vi "to string.vi"(8 "error in":errorcluster, 11 "TDMS datalogger configuration in":refnum<class "TDMS datalogger configuration.lvclass">) -> (0 "error out":errorcluster, 1 "data":string, 2 "version":string, 3 "TDMS datalogger configuration out":refnum<class "TDMS datalogger configuration.lvclass">)   [LabVIEW 2015, in "TDMS datalogger configuration.lvclass"]
doc: "Provides an interface for saving a module configuration to a file or other serialized data source. It is recommended that all children of this class store data in two sets--data required for its own initialization, and any data required for parent initialization--and that each implementation uses the <b>Call Parent Method</b> primitive to serialize parent information."
uses:
  TDMS datalogger configuration.lvclass
  TDMS datalogger configuration.lvclass/TDMS datalogger configuration.ctl
  <vilib>/NI/Tag Bus Module Framework/module configuration/TBM module configuration.lvclass
  <vilib>/NI/Configuration Framework/serializable configuration/NISE_CEF_serializable configuration.lvclass
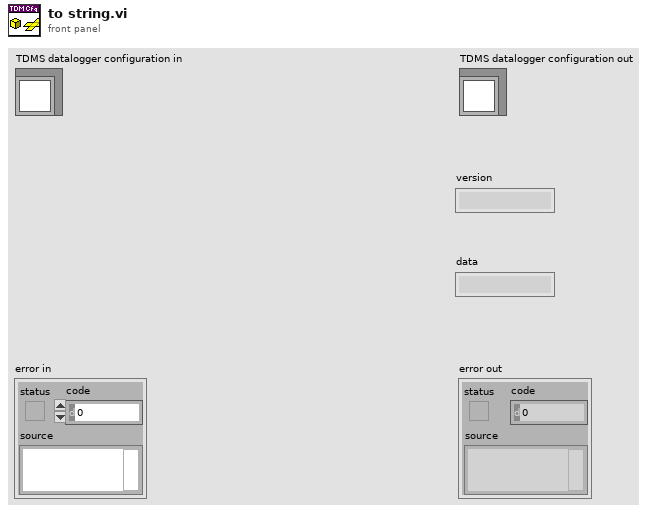
[diagram p1: front panel]
types:
  T1 = typedef "LogRotate.lvclass/options.ctl" = cluster{"max file size (bytes)":i64, "rotate count":u32, "max age (days)":dbl, "No archive dir":bool, "Archive dir":path}
  T2 = typedef "TDMS datalogger configuration.lvclass/Logging Type.ctl" = enum16{"Continuous", "Finite"}
  T3 = typedef "TDMS datalogger configuration.lvclass/Trigger Type.ctl" = enum16{"None", "Start"}
  T4 = typedef "TDMS datalogger configuration.lvclass/Edge Direction.ctl" = enum16{"Rising", "Falling"}
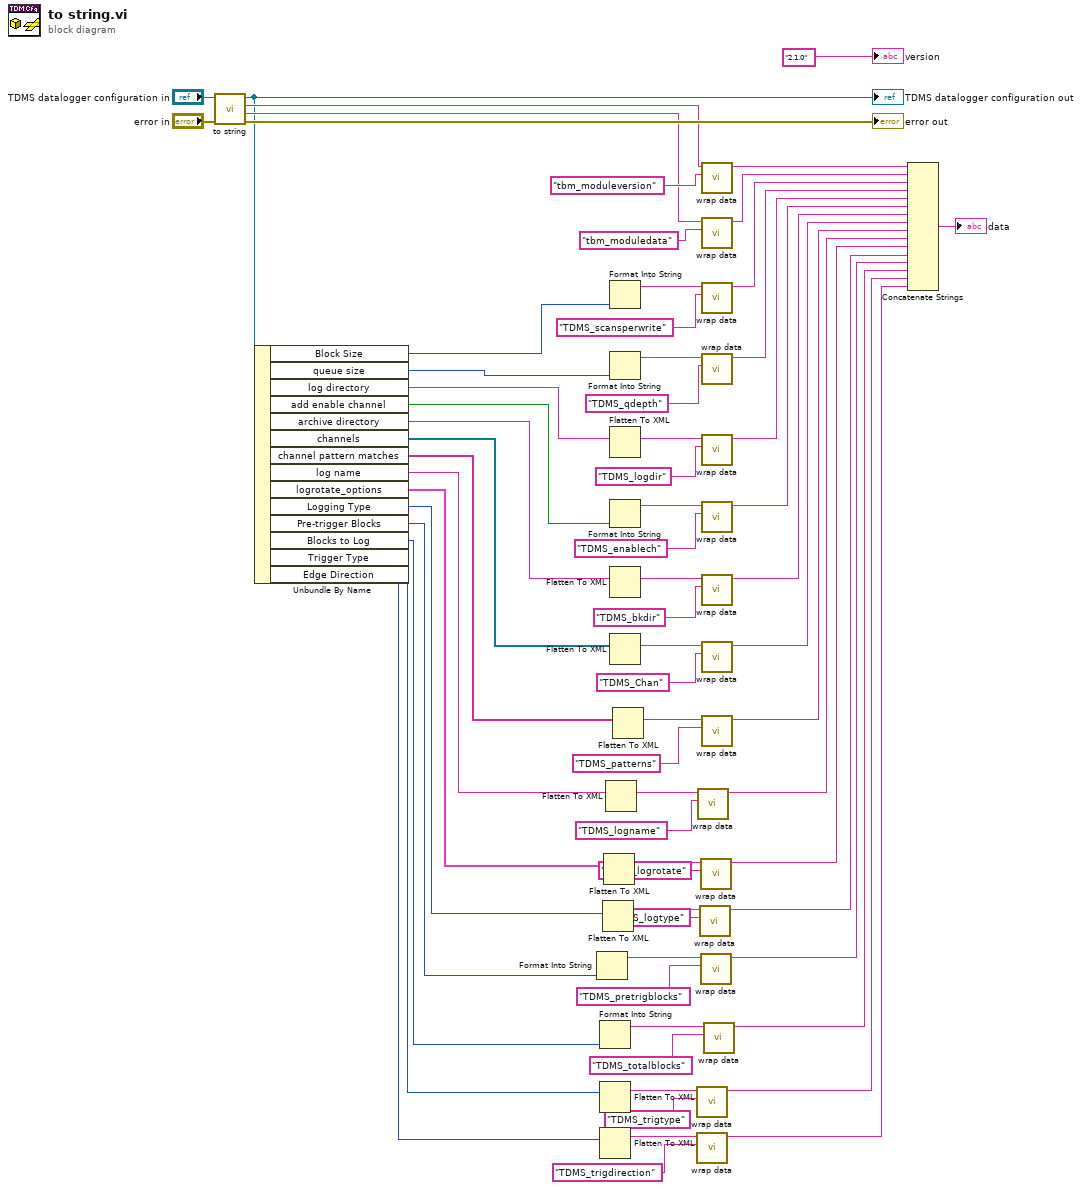
[diagram p0: block diagram]
diagram:
  n1 = call-parent "to string.vi"("error in"="error in", "module configuration in"="TDMS datalogger configuration in") -> ("error out"=→"error out":errorcluster, "data"=w62:string, "version"=w63:string, "module configuration out"=w58:refnum<class "TDMS datalogger configuration.lvclass">)  [unwired: 6 in]
  "TDMS datalogger configuration out" <- w58
  n2 = Unbundle By Name(w58) -> ("Block Size"=w54:u16, "queue size"=w55:u16, "log directory"=w30:string, "add enable channel"=w56:bool, "archive directory"=w29:string, "channels"=w57:refnum<class "TBM channel.lvclass">[], "channel pattern matches"=w35:string[], "log name"=w26:string, "logrotate_options"=w24:T1, "Logging Type"=w18:T2, "Pre-trigger Blocks"=w15:i32, "Blocks to Log"=w12:i32, "Trigger Type"=w9:T3, "Edge Direction"=w6:T4)
  n3 = Format Into String(w15) -> (resulting string=w16:string)  [unwired: 3 in, 1 out]
  n4 = Format Into String(w12) -> (resulting string=w14:string)  [unwired: 3 in, 1 out]
  n5 = Flatten To XML(anything=w9) -> (xml string=w11:string)
  n6 = Flatten To XML(anything=w6) -> (xml string=w8:string)
  n7 = Flatten To XML(anything=w18) -> (xml string=w19:string)
  n8 = Flatten To XML(anything=w24) -> (xml string=w23:string)
  n9 = Flatten To XML(anything=w26) -> (xml string=w27:string)
  n10 = Format Into String(w54) -> (resulting string=w53:string)  [unwired: 3 in, 1 out]
  n11 = Format Into String(w55) -> (resulting string=w51:string)  [unwired: 3 in, 1 out]
  n12 = Flatten To XML(anything=w30) -> (xml string=w49:string)
  n13 = Format Into String(w56) -> (resulting string=w48:string)  [unwired: 3 in, 1 out]
  n14 = Flatten To XML(anything=w29) -> (xml string=w47:string)
  n15 = Flatten To XML(anything=w57) -> (xml string=w46:string)
  n16 = Flatten To XML(anything=w35) -> (xml string=w34:string)
  n17 = call <vilib>:"wrap data.vi"("identifier"="TDMS_trigtype", "data to wrap"=w11) -> ("wrapped data"=w2:string)  [unwired: 9 in]
  n18 = call <vilib>:"wrap data.vi"("identifier"="TDMS_trigdirection", "data to wrap"=w8) -> ("wrapped data"=w1:string)  [unwired: 9 in]
  n19 = call <vilib>:"wrap data.vi"("identifier"="TDMS_logname" ("additional identifier"), "data to wrap"=w27) -> ("wrapped data"=w25:string)  [unwired: 9 in]
  n20 = call <vilib>:"wrap data.vi"("identifier"="TDMS_logtype", "data to wrap"=w19) -> ("wrapped data"=w5:string)  [unwired: 9 in]
  n21 = call <vilib>:"wrap data.vi"("identifier"="TDMS_logrotate", "data to wrap"=w23) -> ("wrapped data"=w21:string)  [unwired: 9 in]
  n22 = call <vilib>:"wrap data.vi"("identifier"="TDMS_pretrigblocks", "data to wrap"=w16) -> ("wrapped data"=w4:string)  [unwired: 9 in]
  n23 = call <vilib>:"wrap data.vi"("identifier"="tbm_moduleversion" ("additional identifier"), "data to wrap"=w63) -> ("wrapped data"=w61:string)  [unwired: 9 in]
  n24 = call <vilib>:"wrap data.vi"("identifier"="tbm_moduledata" ("additional identifier"), "data to wrap"=w62) -> ("wrapped data"=w59:string)  [unwired: 9 in]
  n25 = call <vilib>:"wrap data.vi"("identifier"="TDMS_scansperwrite" ("additional identifier"), "data to wrap"=w53) -> ("wrapped data"=w52:string)  [unwired: 9 in]
  n26 = call <vilib>:"wrap data.vi"("identifier"="TDMS_qdepth" ("additional identifier"), "data to wrap"=w51) -> ("wrapped data"=w50:string)  [unwired: 9 in]
  n27 = call <vilib>:"wrap data.vi"("identifier"="TDMS_logdir" ("additional identifier"), "data to wrap"=w49) -> ("wrapped data"=w45:string)  [unwired: 9 in]
  n28 = call <vilib>:"wrap data.vi"("identifier"="TDMS_enablech" ("additional identifier"), "data to wrap"=w48) -> ("wrapped data"=w44:string)  [unwired: 9 in]
  n29 = call <vilib>:"wrap data.vi"("identifier"="TDMS_bkdir" ("additional identifier"), "data to wrap"=w47) -> ("wrapped data"=w43:string)  [unwired: 9 in]
  n30 = call <vilib>:"wrap data.vi"("identifier"="TDMS_Chan" ("additional identifier"), "data to wrap"=w46) -> ("wrapped data"=w42:string)  [unwired: 9 in]
  n31 = call <vilib>:"wrap data.vi"("identifier"="TDMS_patterns", "data to wrap"=w34) -> ("wrapped data"=w32:string)  [unwired: 9 in]
  n32 = call <vilib>:"wrap data.vi"("identifier"="TDMS_totalblocks", "data to wrap"=w14) -> ("wrapped data"=w3:string)  [unwired: 9 in]
  n33 = Concatenate Strings(w61, w59, w52, w50, w45, w44, w43, w42, w32, w25, w21, w5, w4, w3, w2, w1) -> (→"data":string)
  "version" <- "2.1.0" ("current version")
